vi "Patch data preview initialise-Close TDMS refs.vi"(8 "error in":errorcluster) -> (0 "error out (no error)":errorcluster)   [LabVIEW 2017]
uses:
  Typedefs/Read Write Enum.ctl
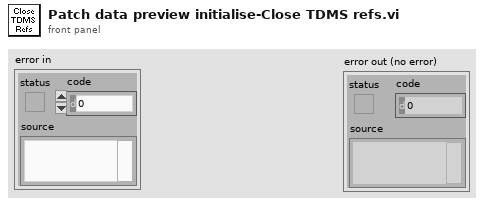
[diagram p1: front panel]
types:
  T1 = typedef "Read Write Enum.ctl" = enum16{"Read", "Write"}
  T2 = typedef "Patch viewer internal cluster.ctl" = cluster{"Image ref":T3, "Coordinates of montage positions":cluster{"X\n\nY":i32[]}[], "TDMS refs":refnum<k34>[], "Frames info":cluster{"Frame numbers used":i32[], "Frame position index":i32[]}, "Number of trials":i32, "Cycles in single trial":i32, "Total number of cycles":i32, "Number of patches":i32, "Pixels in a cycle":i32, "Patches info array":cluster{"Pixels in a patch":i32, "X size of patch":i32, "Y size of patch":i32}[], "error":errorcluster}
  T3 = typedef "IMAQ Image.ctl" = refnum<image>
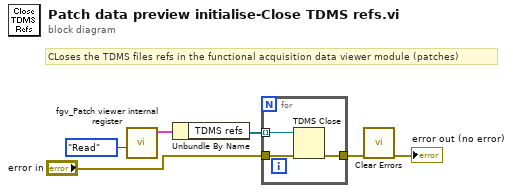
[diagram p0: block diagram]
diagram:
  # "CLoses the TDMS files refs in the functional acquisition data viewer module (patches)"
  n1 = call "fgv_Patch viewer internal register.vi"("Function"=Read_Write_Enum."Read") -> ("Registered setup"=w2:T2)  [unwired: 10 in]
  n2 = Unbundle By Name(w2) -> ("TDMS refs"=w6:refnum<k34>[])
  n3 = for {
    tunnel: w6 -> [w9] mode=indexing
    tunnel: [w8] -> w5
    tunnel: "error in" -> [w7]
    n4 = TDMS Close(8:w7, 11:w9) -> (0:w8:errorcluster)  [unwired: 1 out]
  }
  n5 = call <vilib>:"Clear Errors.vi"("error in (no error)"=w5) -> ("error out"=→"error out (no error)":errorcluster)  [unwired: 5 in, 1 out]
